vi "Lab Panel V4.90.vi"() -> ()   [LabVIEW 2013] (continued)
                    n1117 = Greater Or Equal?(x=w2162, y=w2155) -> (x >= y?=w2164:bool)
                    n1118 = case shown="True" w2164 {
                      tunnel: w2159 -> [w2174 _]
                      tunnel: w2158 -> [w2173 _]
                      tunnel: w2157 -> [w2172 _]
                      tunnel: w2156 -> [w2171 _]
                      frame True {
                        n1119 = stacked-sequence {
                          tunnel: w2174 -> [w2178 _]
                          tunnel: w2173 -> [w2176 w2182]
                          tunnel: w2172 -> [_ w2185]
                          tunnel: w2171 -> [w2175 _]
                          frame #0 {
                            n1120 = Build Array(w2176) -> (w2179:string[])
                            n1121 = Build Array(w2178) -> (w2177:dbl[])
                            n1122 = TDMS Write(0:w2175, 5:"TEST PASS", 7:w2179, 9:w2177) -> (15:w2181:errorcluster)  [unwired: 2 in, 3 out]
                            n1123 = local write "data file error"(w2181) -> ()
                          }
                          frame #1 {
                            n1124 = Bundle(cluster=w2185, "STATUS"=w2182) -> (w2183:T4)  [unwired: 2 in]
                            n1125 = local write "RESULT LAB02-1"(TRUE) -> ()
                            n1126 = local write "DISP LAB02-1"(w2183) -> ()
                          }
                        }
                      }
                      frame False {
                      }
                    }
                  }
                }
              }
              frame #3 {
                # "LAB02-2"
                n1127 = Less?(x=w2186, y=2) -> (x < y?=w2189:bool)
                n1128 = local read "DISP LAB02-2"() -> (w2191:T4)
                n1129 = Unbundle(w2191) -> ("STATUS"=w2192:string)  [unwired: 2 out]
                n1130 = Equal?(x=w2192, y="RUN") -> (x = y?=w2188:bool)
                n1131 = And(x=w2188, y=w2189) -> (x .and. y?=w2187:bool)
                n1132 = case shown="True" w2187 {
                  tunnel: w2191 -> [_ w2197]
                  tunnel: w2186 -> [_ w2201]
                  frame False {
                  }
                  frame True {
                    n1133 = local read "SET LAB02-2"() -> (w2203:T5)
                    n1134 = local read "TDMS LAB02-2"() -> (w2196:refnum<k34>)
                    n1135 = Unbundle(w2197) -> ("CYCLE"=w2202:dbl)  [unwired: 2 out]
                    n1136 = Unbundle(w2203) -> ("CYCLES"=w2194:dbl, "T-RISE mins"=w2200:dbl)  [unwired: 3 out]
                    n1137 = case shown="\"T-RISE TEST\"" w2201 {
                      tunnel: w2200 -> [_ _ w2210]
                      tunnel: [w2205 w2207 w2210] -> w2199
                      tunnel: w2194 -> [w2205 w2207 _]
                      tunnel: ["CHART PASS" "CYCLE PASS" "T-RISE PASS"] -> w2198
                      frame "CHART TEST", Default {
                      }
                      frame "CYCLE TEST" {
                      }
                      frame "T-RISE TEST" {
                      }
                    }
                    n1138 = Increment(x=w2194) -> (x+1=w2195:dbl)
                    n1139 = Greater Or Equal?(x=w2202, y=w2195) -> (x >= y?=w2204:bool)
                    n1140 = case shown="True" w2204 {
                      tunnel: w2199 -> [w2214 _]
                      tunnel: w2198 -> [w2213 _]
                      tunnel: w2197 -> [w2212 _]
                      tunnel: w2196 -> [w2211 _]
                      frame True {
                        n1141 = stacked-sequence {
                          tunnel: w2214 -> [w2218 _]
                          tunnel: w2213 -> [w2216 w2222]
                          tunnel: w2212 -> [_ w2225]
                          tunnel: w2211 -> [w2215 _]
                          frame #0 {
                            n1142 = Build Array(w2216) -> (w2219:string[])
                            n1143 = Build Array(w2218) -> (w2217:dbl[])
                            n1144 = TDMS Write(0:w2215, 5:"TEST PASS", 7:w2219, 9:w2217) -> (15:w2221:errorcluster)  [unwired: 2 in, 3 out]
                            n1145 = local write "data file error"(w2221) -> ()
                          }
                          frame #1 {
                            n1146 = Bundle(cluster=w2225, "STATUS"=w2222) -> (w2223:T4)  [unwired: 2 in]
                            n1147 = local write "RESULT LAB02-2"(TRUE) -> ()
                            n1148 = local write "DISP LAB02-2"(w2223) -> ()
                          }
                        }
                      }
                      frame False {
                      }
                    }
                  }
                }
              }
              frame #4 {
                # "LAB03-1"
                n1149 = Less?(x=w2226, y=2) -> (x < y?=w2229:bool)
                n1150 = local read "DISP LAB03-1"() -> (w2231:T4)
                n1151 = Unbundle(w2231) -> ("STATUS"=w2232:string)  [unwired: 2 out]
                n1152 = Equal?(x=w2232, y="RUN") -> (x = y?=w2228:bool)
                n1153 = And(x=w2228, y=w2229) -> (x .and. y?=w2227:bool)
                n1154 = case shown="True" w2227 {
                  tunnel: w2231 -> [_ w2237]
                  tunnel: w2226 -> [_ w2241]
                  frame False {
                  }
                  frame True {
                    n1155 = local read "SET LAB03-1"() -> (w2243:T5)
                    n1156 = local read "TDMS LAB03-1"() -> (w2236:refnum<k34>)
                    n1157 = Unbundle(w2237) -> ("CYCLE"=w2242:dbl)  [unwired: 2 out]
                    n1158 = Unbundle(w2243) -> ("CYCLES"=w2234:dbl, "T-RISE mins"=w2240:dbl)  [unwired: 3 out]
                    n1159 = case shown="\"T-RISE TEST\"" w2241 {
                      tunnel: w2240 -> [_ _ w2250]
                      tunnel: [w2245 w2247 w2250] -> w2239
                      tunnel: w2234 -> [w2245 w2247 _]
                      tunnel: ["CHART PASS" "CYCLE PASS" "T-RISE PASS"] -> w2238
                      frame "CHART TEST", Default {
                      }
                      frame "CYCLE TEST" {
                      }
                      frame "T-RISE TEST" {
                      }
                    }
                    n1160 = Increment(x=w2234) -> (x+1=w2235:dbl)
                    n1161 = Greater Or Equal?(x=w2242, y=w2235) -> (x >= y?=w2244:bool)
                    n1162 = case shown="True" w2244 {
                      tunnel: w2239 -> [w2254 _]
                      tunnel: w2238 -> [w2253 _]
                      tunnel: w2237 -> [w2252 _]
                      tunnel: w2236 -> [w2251 _]
                      frame True {
                        n1163 = stacked-sequence {
                          tunnel: w2254 -> [w2258 _]
                          tunnel: w2253 -> [w2256 w2262]
                          tunnel: w2252 -> [_ w2265]
                          tunnel: w2251 -> [w2255 _]
                          frame #0 {
                            n1164 = Build Array(w2256) -> (w2259:string[])
                            n1165 = Build Array(w2258) -> (w2257:dbl[])
                            n1166 = TDMS Write(0:w2255, 5:"TEST PASS", 7:w2259, 9:w2257) -> (15:w2261:errorcluster)  [unwired: 2 in, 3 out]
                            n1167 = local write "data file error"(w2261) -> ()
                          }
                          frame #1 {
                            n1168 = Bundle(cluster=w2265, "STATUS"=w2262) -> (w2263:T4)  [unwired: 2 in]
                            n1169 = local write "RESULT LAB03-1"(TRUE) -> ()
                            n1170 = local write "DISP LAB03-1"(w2263) -> ()
                          }
                        }
                      }
                      frame False {
                      }
                    }
                  }
                }
              }
              frame #5 {
                # "LAB03-2"
                n1171 = Less?(x=w2266, y=2) -> (x < y?=w2269:bool)
                n1172 = local read "DISP LAB03-2"() -> (w2271:T4)
                n1173 = Unbundle(w2271) -> ("STATUS"=w2272:string)  [unwired: 2 out]
                n1174 = Equal?(x=w2272, y="RUN") -> (x = y?=w2268:bool)
                n1175 = And(x=w2268, y=w2269) -> (x .and. y?=w2267:bool)
                n1176 = case shown="True" w2267 {
                  tunnel: w2271 -> [_ w2277]
                  tunnel: w2266 -> [_ w2281]
                  frame False {
                  }
                  frame True {
                    n1177 = local read "SET LAB03-2"() -> (w2283:T5)
                    n1178 = local read "TDMS LAB03-2"() -> (w2276:refnum<k34>)
                    n1179 = Unbundle(w2277) -> ("CYCLE"=w2282:dbl)  [unwired: 2 out]
                    n1180 = Unbundle(w2283) -> ("CYCLES"=w2274:dbl, "T-RISE mins"=w2280:dbl)  [unwired: 3 out]
                    n1181 = case shown="\"T-RISE TEST\"" w2281 {
                      tunnel: w2280 -> [_ _ w2290]
                      tunnel: [w2285 w2287 w2290] -> w2279
                      tunnel: w2274 -> [w2285 w2287 _]
                      tunnel: ["CHART PASS" "CYCLE PASS" "T-RISE PASS"] -> w2278
                      frame "CHART TEST", Default {
                      }
                      frame "CYCLE TEST" {
                      }
                      frame "T-RISE TEST" {
                      }
                    }
                    n1182 = Increment(x=w2274) -> (x+1=w2275:dbl)
                    n1183 = Greater Or Equal?(x=w2282, y=w2275) -> (x >= y?=w2284:bool)
                    n1184 = case shown="True" w2284 {
                      tunnel: w2279 -> [w2294 _]
                      tunnel: w2278 -> [w2293 _]
                      tunnel: w2277 -> [w2292 _]
                      tunnel: w2276 -> [w2291 _]
                      frame True {
                        n1185 = stacked-sequence {
                          tunnel: w2294 -> [w2298 _]
                          tunnel: w2293 -> [w2296 w2302]
                          tunnel: w2292 -> [_ w2305]
                          tunnel: w2291 -> [w2295 _]
                          frame #0 {
                            n1186 = Build Array(w2296) -> (w2299:string[])
                            n1187 = Build Array(w2298) -> (w2297:dbl[])
                            n1188 = TDMS Write(0:w2295, 5:"TEST PASS", 7:w2299, 9:w2297) -> (15:w2301:errorcluster)  [unwired: 2 in, 3 out]
                            n1189 = local write "data file error"(w2301) -> ()
                          }
                          frame #1 {
                            n1190 = Bundle(cluster=w2305, "STATUS"=w2302) -> (w2303:T4)  [unwired: 2 in]
                            n1191 = local write "RESULT LAB03-2"(TRUE) -> ()
                            n1192 = local write "DISP LAB03-2"(w2303) -> ()
                          }
                        }
                      }
                      frame False {
                      }
                    }
                  }
                }
              }
              frame #6 {
                # "LAB04-1"
                n1193 = Less?(x=w2306, y=2) -> (x < y?=w2309:bool)
                n1194 = local read "DISP LAB04-1"() -> (w2311:T4)
                n1195 = Unbundle(w2311) -> ("STATUS"=w2312:string)  [unwired: 2 out]
                n1196 = Equal?(x=w2312, y="RUN") -> (x = y?=w2308:bool)
                n1197 = And(x=w2308, y=w2309) -> (x .and. y?=w2307:bool)
                n1198 = case shown="True" w2307 {
                  tunnel: w2311 -> [_ w2317]
                  tunnel: w2306 -> [_ w2321]
                  frame False {
                  }
                  frame True {
                    n1199 = local read "SET LAB04-1"() -> (w2323:T5)
                    n1200 = local read "TDMS LAB04-1"() -> (w2316:refnum<k34>)
                    n1201 = Unbundle(w2317) -> ("CYCLE"=w2322:dbl)  [unwired: 2 out]
                    n1202 = Unbundle(w2323) -> ("CYCLES"=w2314:dbl, "T-RISE mins"=w2320:dbl)  [unwired: 3 out]
                    n1203 = case shown="\"T-RISE TEST\"" w2321 {
                      tunnel: w2320 -> [_ _ w2330]
                      tunnel: [w2325 w2327 w2330] -> w2319
                      tunnel: w2314 -> [w2325 w2327 _]
                      tunnel: ["CHART PASS" "CYCLE PASS" "T-RISE PASS"] -> w2318
                      frame "CHART TEST", Default {
                      }
                      frame "CYCLE TEST" {
                      }
                      frame "T-RISE TEST" {
                      }
                    }
                    n1204 = Increment(x=w2314) -> (x+1=w2315:dbl)
                    n1205 = Greater Or Equal?(x=w2322, y=w2315) -> (x >= y?=w2324:bool)
                    n1206 = case shown="True" w2324 {
                      tunnel: w2319 -> [w2334 _]
                      tunnel: w2318 -> [w2333 _]
                      tunnel: w2317 -> [w2332 _]
                      tunnel: w2316 -> [w2331 _]
                      frame True {
                        n1207 = stacked-sequence {
                          tunnel: w2334 -> [w2338 _]
                          tunnel: w2333 -> [w2336 w2342]
                          tunnel: w2332 -> [_ w2345]
                          tunnel: w2331 -> [w2335 _]
                          frame #0 {
                            n1208 = Build Array(w2336) -> (w2339:string[])
                            n1209 = Build Array(w2338) -> (w2337:dbl[])
                            n1210 = TDMS Write(0:w2335, 5:"TEST PASS", 7:w2339, 9:w2337) -> (15:w2341:errorcluster)  [unwired: 2 in, 3 out]
                            n1211 = local write "data file error"(w2341) -> ()
                          }
                          frame #1 {
                            n1212 = Bundle(cluster=w2345, "STATUS"=w2342) -> (w2343:T4)  [unwired: 2 in]
                            n1213 = local write "RESULT LAB04-1"(TRUE) -> ()
                            n1214 = local write "DISP LAB04-1"(w2343) -> ()
                          }
                        }
                      }
                      frame False {
                      }
                    }
                  }
                }
              }
              frame #7 {
                # "LAB04-2"
                n1215 = Less?(x=w2346, y=2) -> (x < y?=w2349:bool)
                n1216 = local read "DISP LAB04-2"() -> (w2351:T4)
                n1217 = Unbundle(w2351) -> ("STATUS"=w2352:string)  [unwired: 2 out]
                n1218 = Equal?(x=w2352, y="RUN") -> (x = y?=w2348:bool)
                n1219 = And(x=w2348, y=w2349) -> (x .and. y?=w2347:bool)
                n1220 = case shown="True" w2347 {
                  tunnel: w2351 -> [_ w2357]
                  tunnel: w2346 -> [_ w2361]
                  frame False {
                  }
                  frame True {
                    n1221 = local read "SET LAB04-2"() -> (w2363:T5)
                    n1222 = local read "TDMS LAB04-2"() -> (w2356:refnum<k34>)
                    n1223 = Unbundle(w2357) -> ("CYCLE"=w2362:dbl)  [unwired: 2 out]
                    n1224 = Unbundle(w2363) -> ("CYCLES"=w2354:dbl, "T-RISE mins"=w2360:dbl)  [unwired: 3 out]
                    n1225 = case shown="\"T-RISE TEST\"" w2361 {
                      tunnel: w2360 -> [_ _ w2370]
                      tunnel: [w2365 w2367 w2370] -> w2359
                      tunnel: w2354 -> [w2365 w2367 _]
                      tunnel: ["CHART PASS" "CYCLE PASS" "T-RISE PASS"] -> w2358
                      frame "CHART TEST", Default {
                      }
                      frame "CYCLE TEST" {
                      }
                      frame "T-RISE TEST" {
                      }
                    }
                    n1226 = Increment(x=w2354) -> (x+1=w2355:dbl)
                    n1227 = Greater Or Equal?(x=w2362, y=w2355) -> (x >= y?=w2364:bool)
                    n1228 = case shown="True" w2364 {
                      tunnel: w2359 -> [w2374 _]
                      tunnel: w2358 -> [w2373 _]
                      tunnel: w2357 -> [w2372 _]
                      tunnel: w2356 -> [w2371 _]
                      frame True {
                        n1229 = stacked-sequence {
                          tunnel: w2374 -> [w2378 _]
                          tunnel: w2373 -> [w2376 w2382]
                          tunnel: w2372 -> [_ w2385]
                          tunnel: w2371 -> [w2375 _]
                          frame #0 {
                            n1230 = Build Array(w2376) -> (w2379:string[])
                            n1231 = Build Array(w2378) -> (w2377:dbl[])
                            n1232 = TDMS Write(0:w2375, 5:"TEST PASS", 7:w2379, 9:w2377) -> (15:w2381:errorcluster)  [unwired: 2 in, 3 out]
                            n1233 = local write "data file error"(w2381) -> ()
                          }
                          frame #1 {
                            n1234 = Bundle(cluster=w2385, "STATUS"=w2382) -> (w2383:T4)  [unwired: 2 in]
                            n1235 = local write "RESULT LAB04-2"(TRUE) -> ()
                            n1236 = local write "DISP LAB04-2"(w2383) -> ()
                          }
                        }
                      }
                      frame False {
                      }
                    }
                  }
                }
              }
              frame #8 {
                # "LAB05-1"
                n1237 = Less?(x=w2386, y=2) -> (x < y?=w2389:bool)
                n1238 = local read "DISP LAB05-1"() -> (w2391:T4)
                n1239 = Unbundle(w2391) -> ("STATUS"=w2392:string)  [unwired: 2 out]
                n1240 = Equal?(x=w2392, y="RUN") -> (x = y?=w2388:bool)
                n1241 = And(x=w2388, y=w2389) -> (x .and. y?=w2387:bool)
                n1242 = case shown="True" w2387 {
                  tunnel: w2391 -> [_ w2397]
                  tunnel: w2386 -> [_ w2401]
                  frame False {
                  }
                  frame True {
                    n1243 = local read "SET LAB05-1"() -> (w2403:T5)
                    n1244 = local read "TDMS LAB05-1"() -> (w2396:refnum<k34>)
                    n1245 = Unbundle(w2397) -> ("CYCLE"=w2402:dbl)  [unwired: 2 out]
                    n1246 = Unbundle(w2403) -> ("CYCLES"=w2394:dbl, "T-RISE mins"=w2400:dbl)  [unwired: 3 out]
                    n1247 = case shown="\"T-RISE TEST\"" w2401 {
                      tunnel: w2400 -> [_ _ w2410]
                      tunnel: [w2405 w2407 w2410] -> w2399
                      tunnel: w2394 -> [w2405 w2407 _]
                      tunnel: ["CHART PASS" "CYCLE PASS" "T-RISE PASS"] -> w2398
                      frame "CHART TEST", Default {
                      }
                      frame "CYCLE TEST" {
                      }
                      frame "T-RISE TEST" {
                      }
                    }
                    n1248 = Increment(x=w2394) -> (x+1=w2395:dbl)
                    n1249 = Greater Or Equal?(x=w2402, y=w2395) -> (x >= y?=w2404:bool)
                    n1250 = case shown="True" w2404 {
                      tunnel: w2399 -> [w2414 _]
                      tunnel: w2398 -> [w2413 _]
                      tunnel: w2397 -> [w2412 _]
                      tunnel: w2396 -> [w2411 _]
                      frame True {
                        n1251 = stacked-sequence {
                          tunnel: w2414 -> [w2418 _]
                          tunnel: w2413 -> [w2416 w2422]
                          tunnel: w2412 -> [_ w2425]
                          tunnel: w2411 -> [w2415 _]
                          frame #0 {
                            n1252 = Build Array(w2416) -> (w2419:string[])
                            n1253 = Build Array(w2418) -> (w2417:dbl[])
                            n1254 = TDMS Write(0:w2415, 5:"TEST PASS", 7:w2419, 9:w2417) -> (15:w2421:errorcluster)  [unwired: 2 in, 3 out]
                            n1255 = local write "data file error"(w2421) -> ()
                          }
                          frame #1 {
                            n1256 = Bundle(cluster=w2425, "STATUS"=w2422) -> (w2423:T4)  [unwired: 2 in]
                            n1257 = local write "RESULT LAB05-1"(TRUE) -> ()
                            n1258 = local write "DISP LAB05-1"(w2423) -> ()
                          }
                        }
                      }
                      frame False {
                      }
                    }
                  }
                }
              }
              frame #9 {
                # "LAB05-2"
                n1259 = Less?(x=w2426, y=2) -> (x < y?=w2429:bool)
                n1260 = local read "DISP LAB05-2"() -> (w2431:T4)
                n1261 = Unbundle(w2431) -> ("STATUS"=w2432:string)  [unwired: 2 out]
                n1262 = Equal?(x=w2432, y="RUN") -> (x = y?=w2428:bool)
                n1263 = And(x=w2428, y=w2429) -> (x .and. y?=w2427:bool)
                n1264 = case shown="True" w2427 {
                  tunnel: w2431 -> [_ w2437]
                  tunnel: w2426 -> [_ w2441]
                  frame False {
                  }
                  frame True {
                    n1265 = local read "SET LAB05-2"() -> (w2443:T5)
                    n1266 = local read "TDMS LAB05-2"() -> (w2436:refnum<k34>)
                    n1267 = Unbundle(w2437) -> ("CYCLE"=w2442:dbl)  [unwired: 2 out]
                    n1268 = Unbundle(w2443) -> ("CYCLES"=w2434:dbl, "T-RISE mins"=w2440:dbl)  [unwired: 3 out]
                    n1269 = case shown="\"T-RISE TEST\"" w2441 {
                      tunnel: w2440 -> [_ _ w2450]
                      tunnel: [w2445 w2447 w2450] -> w2439
                      tunnel: w2434 -> [w2445 w2447 _]
                      tunnel: ["CHART PASS" "CYCLE PASS" "T-RISE PASS"] -> w2438
                      frame "CHART TEST", Default {
                      }
                      frame "CYCLE TEST" {
                      }
                      frame "T-RISE TEST" {
                      }
                    }
                    n1270 = Increment(x=w2434) -> (x+1=w2435:dbl)
                    n1271 = Greater Or Equal?(x=w2442, y=w2435) -> (x >= y?=w2444:bool)
                    n1272 = case shown="True" w2444 {
                      tunnel: w2439 -> [w2454 _]
                      tunnel: w2438 -> [w2453 _]
                      tunnel: w2437 -> [w2452 _]
                      tunnel: w2436 -> [w2451 _]
                      frame True {
                        n1273 = stacked-sequence {
                          tunnel: w2454 -> [w2458 _]
                          tunnel: w2453 -> [w2456 w2462]
                          tunnel: w2452 -> [_ w2465]
                          tunnel: w2451 -> [w2455 _]
                          frame #0 {
                            n1274 = Build Array(w2456) -> (w2459:string[])
                            n1275 = Build Array(w2458) -> (w2457:dbl[])
                            n1276 = TDMS Write(0:w2455, 5:"TEST PASS", 7:w2459, 9:w2457) -> (15:w2461:errorcluster)  [unwired: 2 in, 3 out]
                            n1277 = local write "data file error"(w2461) -> ()
                          }
                          frame #1 {
                            n1278 = Bundle(cluster=w2465, "STATUS"=w2462) -> (w2463:T4)  [unwired: 2 in]
                            n1279 = local write "RESULT LAB05-2"(TRUE) -> ()
                            n1280 = local write "DISP LAB05-2"(w2463) -> ()
                          }
                        }
                      }
                      frame False {
                      }
                    }
                  }
                }
              }
            }
          }
          frame #5 {
            # "check if test cycles reached for temperature rise test"
            n1281 = stacked-sequence {
              tunnel: w2495 -> [_ _ _ _ _ _ _ _ _ _]
              tunnel: w2494 -> [_ _ _ _ _ _ _ _ _ _]
              tunnel: w2493 -> [_ _ _ _ _ _ _ _ _ _]
              tunnel: w2492 -> [_ _ _ _ _ _ _ _ _ _]
              tunnel: w2491 -> [_ _ _ _ _ _ _ _ _ _]
              tunnel: w2490 -> [_ _ _ _ _ _ _ _ _ _]
              tunnel: w2489 -> [_ _ _ _ _ _ _ _ _ _]
              tunnel: w2488 -> [_ _ _ _ _ _ _ _ _ _]
              tunnel: w2487 -> [_ _ _ _ _ _ _ _ _ _]
              tunnel: w2486 -> [_ _ _ _ _ _ _ _ _ _]
              tunnel: w2485 -> [w2501 _ _ _ _ _ _ _ _ _]
              tunnel: w2475 -> [w2496 _ _ _ _ _ _ _ _ _]
              tunnel: w2484 -> [_ w2527 _ _ _ _ _ _ _ _]
              tunnel: w2483 -> [_ _ w2557 _ _ _ _ _ _ _]
              tunnel: w2482 -> [_ _ _ w2587 _ _ _ _ _ _]
              tunnel: w2481 -> [_ _ _ _ w2617 _ _ _ _ _]
              tunnel: w2480 -> [_ _ _ _ _ w2647 _ _ _ _]
              tunnel: w2479 -> [_ _ _ _ _ _ w2677 _ _ _]
              tunnel: w2478 -> [_ _ _ _ _ _ _ w2707 _ _]
              tunnel: w2477 -> [_ _ _ _ _ _ _ _ w2737 _]
              tunnel: w2476 -> [_ _ _ _ _ _ _ _ _ w2767]
              tunnel: w2474 -> [_ w2526 _ _ _ _ _ _ _ _]
              tunnel: w2473 -> [_ _ w2556 _ _ _ _ _ _ _]
              tunnel: w2472 -> [_ _ _ w2586 _ _ _ _ _ _]
              tunnel: w2471 -> [_ _ _ _ w2616 _ _ _ _ _]
              tunnel: w2470 -> [_ _ _ _ _ w2646 _ _ _ _]
              tunnel: w2469 -> [_ _ _ _ _ _ w2676 _ _ _]
              tunnel: w2468 -> [_ _ _ _ _ _ _ w2706 _ _]
              tunnel: w2467 -> [_ _ _ _ _ _ _ _ w2736 _]
              tunnel: w2466 -> [_ _ _ _ _ _ _ _ _ w2766]
              frame #0 {
                # "LAB01-1"
                n1282 = Equal?(x=w2501, y=2) -> (x = y?=w2499:bool)
                n1283 = local read "DISP LAB01-1"() -> (w2502:T4)
                n1284 = Unbundle(w2502) -> ("STATUS"=w2503:string)  [unwired: 2 out]
                n1285 = Equal?(x=w2503, y="RUN") -> (x = y?=w2498:bool)
                n1286 = And(x=w2498, y=w2499) -> (x .and. y?=w2497:bool)
                n1287 = case shown="True" w2497 {
                  tunnel: w2502 -> [_ w2506]
                  tunnel: w2496 -> [_ w2509]
                  frame False {
                  }
                  frame True {
                    n1288 = local read "SET LAB01-1"() -> (w2508:T5)
                    n1289 = local read "TDMS LAB01-1"() -> (w2505:refnum<k34>)
                    n1290 = Unbundle(w2506) -> ("CYCLE"=w2510:dbl)  [unwired: 2 out]
                    n1291 = Unbundle(w2508) -> ("T-RISE mins"=w2507:dbl)  [unwired: 4 out]
                    n1292 = Greater Or Equal?(x=w2510, y=w2509) -> (x >= y?=w2511:bool)
                    n1293 = case shown="True" w2511 {
                      tunnel: w2507 -> [w2514 _]
                      tunnel: w2506 -> [w2513 _]
                      tunnel: w2505 -> [w2512 _]
                      frame True {
                        n1294 = stacked-sequence {
                          tunnel: w2514 -> [w2517 _]
                          tunnel: w2513 -> [_ w2522]
                          tunnel: w2512 -> [w2515 _]
                          frame #0 {
                            n1295 = Build Array("T-RISE") -> (w2519:string[])
                            n1296 = Build Array(w2517) -> (w2518:dbl[])
                            n1297 = TDMS Write(0:w2515, 5:"TEST PASS", 7:w2519, 9:w2518) -> (15:w2521:errorcluster)  [unwired: 2 in, 3 out]
                            n1298 = local write "data file error"(w2521) -> ()
                          }
                          frame #1 {
                            n1299 = Bundle(cluster=w2522, "STATUS"="T-RISE PASS") -> (w2524:T4)  [unwired: 2 in]
                            n1300 = local write "RESULT LAB01-1"(TRUE) -> ()
                            n1301 = local write "DISP LAB01-1"(w2524) -> ()
                          }
                        }
                      }
                      frame False {
                      }
                    }
                  }
                }
              }
              frame #1 {
                # "LAB01-2"
                n1302 = Equal?(x=w2527, y=2) -> (x = y?=w2530:bool)
                n1303 = local read "DISP LAB01-2"() -> (w2532:T4)
                n1304 = Unbundle(w2532) -> ("STATUS"=w2533:string)  [unwired: 2 out]
                n1305 = Equal?(x=w2533, y="RUN") -> (x = y?=w2529:bool)
                n1306 = And(x=w2529, y=w2530) -> (x .and. y?=w2528:bool)
                n1307 = case shown="True" w2528 {
                  tunnel: w2532 -> [_ w2536]
                  tunnel: w2526 -> [_ w2539]
                  frame False {
                  }
                  frame True {
                    n1308 = local read "SET LAB01-2"() -> (w2538:T5)
                    n1309 = local read "TDMS LAB01-2"() -> (w2535:refnum<k34>)
                    n1310 = Unbundle(w2536) -> ("CYCLE"=w2540:dbl)  [unwired: 2 out]
                    n1311 = Unbundle(w2538) -> ("T-RISE mins"=w2537:dbl)  [unwired: 4 out]
                    n1312 = Greater Or Equal?(x=w2540, y=w2539) -> (x >= y?=w2541:bool)
                    n1313 = case shown="True" w2541 {
                      tunnel: w2537 -> [w2544 _]
                      tunnel: w2536 -> [w2543 _]
                      tunnel: w2535 -> [w2542 _]
                      frame True {
                        n1314 = stacked-sequence {
                          tunnel: w2544 -> [w2547 _]
                          tunnel: w2543 -> [_ w2552]
                          tunnel: w2542 -> [w2545 _]
                          frame #0 {
                            n1315 = Build Array("T-RISE") -> (w2549:string[])
                            n1316 = Build Array(w2547) -> (w2548:dbl[])
                            n1317 = TDMS Write(0:w2545, 5:"TEST PASS", 7:w2549, 9:w2548) -> (15:w2551:errorcluster)  [unwired: 2 in, 3 out]
                            n1318 = local write "data file error"(w2551) -> ()
                          }
                          frame #1 {
                            n1319 = Bundle(cluster=w2552, "STATUS"="T-RISE PASS") -> (w2554:T4)  [unwired: 2 in]
                            n1320 = local write "RESULT LAB01-2"(TRUE) -> ()
                            n1321 = local write "DISP LAB01-2"(w2554) -> ()
                          }
                        }
                      }
                      frame False {
                      }
                    }
                  }
                }
              }
              frame #2 {
                # "LAB02-1"
                n1322 = Equal?(x=w2557, y=2) -> (x = y?=w2560:bool)
                n1323 = local read "DISP LAB02-1"() -> (w2562:T4)
                n1324 = Unbundle(w2562) -> ("STATUS"=w2563:string)  [unwired: 2 out]
                n1325 = Equal?(x=w2563, y="RUN") -> (x = y?=w2559:bool)
                n1326 = And(x=w2559, y=w2560) -> (x .and. y?=w2558:bool)
                n1327 = case shown="True" w2558 {
                  tunnel: w2562 -> [_ w2566]
                  tunnel: w2556 -> [_ w2569]
                  frame False {
                  }
                  frame True {
                    n1328 = local read "SET LAB02-1"() -> (w2568:T5)
                    n1329 = local read "TDMS LAB02-1"() -> (w2565:refnum<k34>)
                    n1330 = Unbundle(w2566) -> ("CYCLE"=w2570:dbl)  [unwired: 2 out]
                    n1331 = Unbundle(w2568) -> ("T-RISE mins"=w2567:dbl)  [unwired: 4 out]
                    n1332 = Greater Or Equal?(x=w2570, y=w2569) -> (x >= y?=w2571:bool)
                    n1333 = case shown="True" w2571 {
                      tunnel: w2567 -> [w2574 _]
                      tunnel: w2566 -> [w2573 _]
                      tunnel: w2565 -> [w2572 _]
                      frame True {
                        n1334 = stacked-sequence {
                          tunnel: w2574 -> [w2577 _]
                          tunnel: w2573 -> [_ w2582]
                          tunnel: w2572 -> [w2575 _]
                          frame #0 {
                            n1335 = Build Array("T-RISE") -> (w2579:string[])
                            n1336 = Build Array(w2577) -> (w2578:dbl[])
                            n1337 = TDMS Write(0:w2575, 5:"TEST PASS", 7:w2579, 9:w2578) -> (15:w2581:errorcluster)  [unwired: 2 in, 3 out]
                            n1338 = local write "data file error"(w2581) -> ()
                          }
                          frame #1 {
                            n1339 = Bundle(cluster=w2582, "STATUS"="T-RISE PASS") -> (w2584:T4)  [unwired: 2 in]
                            n1340 = local write "RESULT LAB02-1"(TRUE) -> ()
                            n1341 = local write "DISP LAB02-1"(w2584) -> ()
                          }
                        }
                      }
                      frame False {
                      }
                    }
                  }
                }
              }
              frame #3 {
                # "LAB02-2"
                n1342 = Equal?(x=w2587, y=2) -> (x = y?=w2590:bool)
                n1343 = local read "DISP LAB02-2"() -> (w2592:T4)
                n1344 = Unbundle(w2592) -> ("STATUS"=w2593:string)  [unwired: 2 out]
                n1345 = Equal?(x=w2593, y="RUN") -> (x = y?=w2589:bool)
                n1346 = And(x=w2589, y=w2590) -> (x .and. y?=w2588:bool)
                n1347 = case shown="True" w2588 {
                  tunnel: w2592 -> [_ w2596]
                  tunnel: w2586 -> [_ w2599]
                  frame False {
                  }
                  frame True {
                    n1348 = local read "SET LAB02-2"() -> (w2598:T5)
                    n1349 = local read "TDMS LAB02-2"() -> (w2595:refnum<k34>)
                    n1350 = Unbundle(w2596) -> ("CYCLE"=w2600:dbl)  [unwired: 2 out]
                    n1351 = Unbundle(w2598) -> ("T-RISE mins"=w2597:dbl)  [unwired: 4 out]
                    n1352 = Greater Or Equal?(x=w2600, y=w2599) -> (x >= y?=w2601:bool)
                    n1353 = case shown="True" w2601 {
                      tunnel: w2597 -> [w2604 _]
                      tunnel: w2596 -> [w2603 _]
                      tunnel: w2595 -> [w2602 _]
                      frame True {
                        n1354 = stacked-sequence {
                          tunnel: w2604 -> [w2607 _]
                          tunnel: w2603 -> [_ w2612]
                          tunnel: w2602 -> [w2605 _]
                          frame #0 {
                            n1355 = Build Array("T-RISE") -> (w2609:string[])
                            n1356 = Build Array(w2607) -> (w2608:dbl[])
                            n1357 = TDMS Write(0:w2605, 5:"TEST PASS", 7:w2609, 9:w2608) -> (15:w2611:errorcluster)  [unwired: 2 in, 3 out]
                            n1358 = local write "data file error"(w2611) -> ()
                          }
                          frame #1 {
                            n1359 = Bundle(cluster=w2612, "STATUS"="T-RISE PASS") -> (w2614:T4)  [unwired: 2 in]
                            n1360 = local write "RESULT LAB02-2"(TRUE) -> ()
                            n1361 = local write "DISP LAB02-2"(w2614) -> ()
                          }
                        }
                      }
                      frame False {
                      }
                    }
                  }
                }
              }
              frame #4 {
                # "LAB03-1"
                n1362 = Equal?(x=w2617, y=2) -> (x = y?=w2620:bool)
                n1363 = local read "DISP LAB03-1"() -> (w2622:T4)
                n1364 = Unbundle(w2622) -> ("STATUS"=w2623:string)  [unwired: 2 out]
                n1365 = Equal?(x=w2623, y="RUN") -> (x = y?=w2619:bool)
                n1366 = And(x=w2619, y=w2620) -> (x .and. y?=w2618:bool)
                n1367 = case shown="True" w2618 {
                  tunnel: w2622 -> [_ w2626]
                  tunnel: w2616 -> [_ w2629]
                  frame False {
                  }
                  frame True {
                    n1368 = local read "SET LAB03-1"() -> (w2628:T5)
                    n1369 = local read "TDMS LAB03-1"() -> (w2625:refnum<k34>)
                    n1370 = Unbundle(w2626) -> ("CYCLE"=w2630:dbl)  [unwired: 2 out]
                    n1371 = Unbundle(w2628) -> ("T-RISE mins"=w2627:dbl)  [unwired: 4 out]
                    n1372 = Greater Or Equal?(x=w2630, y=w2629) -> (x >= y?=w2631:bool)
                    n1373 = case shown="True" w2631 {
                      tunnel: w2627 -> [w2634 _]
                      tunnel: w2626 -> [w2633 _]
                      tunnel: w2625 -> [w2632 _]
                      frame True {
                        n1374 = stacked-sequence {
                          tunnel: w2634 -> [w2637 _]
                          tunnel: w2633 -> [_ w2642]
                          tunnel: w2632 -> [w2635 _]
                          frame #0 {
                            n1375 = Build Array("T-RISE") -> (w2639:string[])
                            n1376 = Build Array(w2637) -> (w2638:dbl[])
                            n1377 = TDMS Write(0:w2635, 5:"TEST PASS", 7:w2639, 9:w2638) -> (15:w2641:errorcluster)  [unwired: 2 in, 3 out]
                            n1378 = local write "data file error"(w2641) -> ()
                          }
                          frame #1 {
                            n1379 = Bundle(cluster=w2642, "STATUS"="T-RISE PASS") -> (w2644:T4)  [unwired: 2 in]
                            n1380 = local write "RESULT LAB03-1"(TRUE) -> ()
                            n1381 = local write "DISP LAB03-1"(w2644) -> ()
                          }
                        }
                      }
                      frame False {
                      }
                    }
                  }
                }
              }
              frame #5 {
                # "LAB03-2"
                n1382 = Equal?(x=w2647, y=2) -> (x = y?=w2650:bool)
                n1383 = local read "DISP LAB03-2"() -> (w2652:T4)
                n1384 = Unbundle(w2652) -> ("STATUS"=w2653:string)  [unwired: 2 out]
                n1385 = Equal?(x=w2653, y="RUN") -> (x = y?=w2649:bool)
                n1386 = And(x=w2649, y=w2650) -> (x .and. y?=w2648:bool)
                n1387 = case shown="True" w2648 {
                  tunnel: w2652 -> [_ w2656]
                  tunnel: w2646 -> [_ w2659]
                  frame False {
                  }
                  frame True {
                    n1388 = local read "SET LAB03-2"() -> (w2658:T5)
                    n1389 = local read "TDMS LAB03-2"() -> (w2655:refnum<k34>)
                    n1390 = Unbundle(w2656) -> ("CYCLE"=w2660:dbl)  [unwired: 2 out]
                    n1391 = Unbundle(w2658) -> ("T-RISE mins"=w2657:dbl)  [unwired: 4 out]
                    n1392 = Greater Or Equal?(x=w2660, y=w2659) -> (x >= y?=w2661:bool)
                    n1393 = case shown="True" w2661 {
                      tunnel: w2657 -> [w2664 _]
                      tunnel: w2656 -> [w2663 _]
                      tunnel: w2655 -> [w2662 _]
                      frame True {
                        n1394 = stacked-sequence {
                          tunnel: w2664 -> [w2667 _]
                          tunnel: w2663 -> [_ w2672]
                          tunnel: w2662 -> [w2665 _]
                          frame #0 {
                            n1395 = Build Array("T-RISE") -> (w2669:string[])
                            n1396 = Build Array(w2667) -> (w2668:dbl[])
                            n1397 = TDMS Write(0:w2665, 5:"TEST PASS", 7:w2669, 9:w2668) -> (15:w2671:errorcluster)  [unwired: 2 in, 3 out]
                            n1398 = local write "data file error"(w2671) -> ()
                          }
                          frame #1 {
                            n1399 = Bundle(cluster=w2672, "STATUS"="T-RISE PASS") -> (w2674:T4)  [unwired: 2 in]
                            n1400 = local write "RESULT LAB03-2"(TRUE) -> ()
                            n1401 = local write "DISP LAB03-2"(w2674) -> ()
                          }
                        }
                      }
                      frame False {
                      }
                    }
                  }
                }
              }
              frame #6 {
                # "LAB04-1"
                n1402 = Equal?(x=w2677, y=2) -> (x = y?=w2680:bool)
                n1403 = local read "DISP LAB04-1"() -> (w2682:T4)
                n1404 = Unbundle(w2682) -> ("STATUS"=w2683:string)  [unwired: 2 out]
                n1405 = Equal?(x=w2683, y="RUN") -> (x = y?=w2679:bool)
                n1406 = And(x=w2679, y=w2680) -> (x .and. y?=w2678:bool)
                n1407 = case shown="True" w2678 {
                  tunnel: w2682 -> [_ w2686]
                  tunnel: w2676 -> [_ w2689]
                  frame False {
                  }
                  frame True {
                    n1408 = local read "SET LAB04-1"() -> (w2688:T5)
                    n1409 = local read "TDMS LAB04-1"() -> (w2685:refnum<k34>)
                    n1410 = Unbundle(w2686) -> ("CYCLE"=w2690:dbl)  [unwired: 2 out]
                    n1411 = Unbundle(w2688) -> ("T-RISE mins"=w2687:dbl)  [unwired: 4 out]
                    n1412 = Greater Or Equal?(x=w2690, y=w2689) -> (x >= y?=w2691:bool)
                    n1413 = case shown="True" w2691 {
                      tunnel: w2687 -> [w2694 _]
                      tunnel: w2686 -> [w2693 _]
                      tunnel: w2685 -> [w2692 _]
                      frame True {
                        n1414 = stacked-sequence {
                          tunnel: w2694 -> [w2697 _]
                          tunnel: w2693 -> [_ w2702]
                          tunnel: w2692 -> [w2695 _]
                          frame #0 {
                            n1415 = Build Array("T-RISE") -> (w2699:string[])
                            n1416 = Build Array(w2697) -> (w2698:dbl[])
                            n1417 = TDMS Write(0:w2695, 5:"TEST PASS", 7:w2699, 9:w2698) -> (15:w2701:errorcluster)  [unwired: 2 in, 3 out]
                            n1418 = local write "data file error"(w2701) -> ()
                          }
                          frame #1 {
                            n1419 = Bundle(cluster=w2702, "STATUS"="T-RISE PASS") -> (w2704:T4)  [unwired: 2 in]
                            n1420 = local write "RESULT LAB04-1"(TRUE) -> ()
                            n1421 = local write "DISP LAB04-1"(w2704) -> ()
                          }
                        }
                      }
                      frame False {
                      }
                    }
                  }
                }
              }
              frame #7 {
                # "LAB04-2"
                n1422 = Equal?(x=w2707, y=2) -> (x = y?=w2710:bool)
                n1423 = local read "DISP LAB04-2"() -> (w2712:T4)
                n1424 = Unbundle(w2712) -> ("STATUS"=w2713:string)  [unwired: 2 out]
                n1425 = Equal?(x=w2713, y="RUN") -> (x = y?=w2709:bool)
                n1426 = And(x=w2709, y=w2710) -> (x .and. y?=w2708:bool)
                n1427 = case shown="True" w2708 {
                  tunnel: w2712 -> [_ w2716]
                  tunnel: w2706 -> [_ w2719]
                  frame False {
                  }
                  frame True {
                    n1428 = local read "SET LAB04-2"() -> (w2718:T5)
                    n1429 = local read "TDMS LAB04-2"() -> (w2715:refnum<k34>)
                    n1430 = Unbundle(w2716) -> ("CYCLE"=w2720:dbl)  [unwired: 2 out]
                    n1431 = Unbundle(w2718) -> ("T-RISE mins"=w2717:dbl)  [unwired: 4 out]
                    n1432 = Greater Or Equal?(x=w2720, y=w2719) -> (x >= y?=w2721:bool)
                    n1433 = case shown="True" w2721 {
                      tunnel: w2717 -> [w2724 _]
                      tunnel: w2716 -> [w2723 _]
                      tunnel: w2715 -> [w2722 _]
                      frame True {
                        n1434 = stacked-sequence {
                          tunnel: w2724 -> [w2727 _]
                          tunnel: w2723 -> [_ w2732]
                          tunnel: w2722 -> [w2725 _]
                          frame #0 {
                            n1435 = Build Array("T-RISE") -> (w2729:string[])
                            n1436 = Build Array(w2727) -> (w2728:dbl[])
                            n1437 = TDMS Write(0:w2725, 5:"TEST PASS", 7:w2729, 9:w2728) -> (15:w2731:errorcluster)  [unwired: 2 in, 3 out]
                            n1438 = local write "data file error"(w2731) -> ()
                          }
                          frame #1 {
                            n1439 = Bundle(cluster=w2732, "STATUS"="T-RISE PASS") -> (w2734:T4)  [unwired: 2 in]
                            n1440 = local write "RESULT LAB04-2"(TRUE) -> ()
                            n1441 = local write "DISP LAB04-2"(w2734) -> ()
                          }
                        }
                      }
                      frame False {
                      }
                    }
                  }
                }
              }
              frame #8 {
                # "LAB05-1"
                n1442 = Equal?(x=w2737, y=2) -> (x = y?=w2740:bool)
                n1443 = local read "DISP LAB05-1"() -> (w2742:T4)
                n1444 = Unbundle(w2742) -> ("STATUS"=w2743:string)  [unwired: 2 out]
                n1445 = Equal?(x=w2743, y="RUN") -> (x = y?=w2739:bool)
                n1446 = And(x=w2739, y=w2740) -> (x .and. y?=w2738:bool)
                n1447 = case shown="True" w2738 {
                  tunnel: w2742 -> [_ w2746]
                  tunnel: w2736 -> [_ w2749]
                  frame False {
                  }
                  frame True {
                    n1448 = local read "SET LAB05-1"() -> (w2748:T5)
                    n1449 = local read "TDMS LAB05-1"() -> (w2745:refnum<k34>)
                    n1450 = Unbundle(w2746) -> ("CYCLE"=w2750:dbl)  [unwired: 2 out]
                    n1451 = Unbundle(w2748) -> ("T-RISE mins"=w2747:dbl)  [unwired: 4 out]
                    n1452 = Greater Or Equal?(x=w2750, y=w2749) -> (x >= y?=w2751:bool)
                    n1453 = case shown="True" w2751 {
                      tunnel: w2747 -> [w2754 _]
                      tunnel: w2746 -> [w2753 _]
                      tunnel: w2745 -> [w2752 _]
                      frame True {
                        n1454 = stacked-sequence {
                          tunnel: w2754 -> [w2757 _]
                          tunnel: w2753 -> [_ w2762]
                          tunnel: w2752 -> [w2755 _]
                          frame #0 {
                            n1455 = Build Array("T-RISE") -> (w2759:string[])
                            n1456 = Build Array(w2757) -> (w2758:dbl[])
                            n1457 = TDMS Write(0:w2755, 5:"TEST PASS", 7:w2759, 9:w2758) -> (15:w2761:errorcluster)  [unwired: 2 in, 3 out]
                            n1458 = local write "data file error"(w2761) -> ()
                          }
                          frame #1 {
                            n1459 = Bundle(cluster=w2762, "STATUS"="T-RISE PASS") -> (w2764:T4)  [unwired: 2 in]
                            n1460 = local write "RESULT LAB05-1"(TRUE) -> ()
                            n1461 = local write "DISP LAB05-1"(w2764) -> ()
                          }
                        }
                      }
                      frame False {
                      }
                    }
                  }
                }
              }
              frame #9 {
                # "LAB05-2"
                n1462 = Equal?(x=w2767, y=2) -> (x = y?=w2770:bool)
                n1463 = local read "DISP LAB05-2"() -> (w2772:T4)
                n1464 = Unbundle(w2772) -> ("STATUS"=w2773:string)  [unwired: 2 out]
                n1465 = Equal?(x=w2773, y="RUN") -> (x = y?=w2769:bool)
                n1466 = And(x=w2769, y=w2770) -> (x .and. y?=w2768:bool)
                n1467 = case shown="True" w2768 {
                  tunnel: w2772 -> [_ w2776]
                  tunnel: w2766 -> [_ w2779]
                  frame False {
                  }
                  frame True {
                    n1468 = local read "SET LAB05-2"() -> (w2778:T5)
                    n1469 = local read "TDMS LAB05-2"() -> (w2775:refnum<k34>)
                    n1470 = Unbundle(w2776) -> ("CYCLE"=w2780:dbl)  [unwired: 2 out]
                    n1471 = Unbundle(w2778) -> ("T-RISE mins"=w2777:dbl)  [unwired: 4 out]
                    n1472 = Greater Or Equal?(x=w2780, y=w2779) -> (x >= y?=w2781:bool)
                    n1473 = case shown="True" w2781 {
                      tunnel: w2777 -> [w2784 _]
                      tunnel: w2776 -> [w2783 _]
                      tunnel: w2775 -> [w2782 _]
                      frame True {
                        n1474 = stacked-sequence {
                          tunnel: w2784 -> [w2787 _]
                          tunnel: w2783 -> [_ w2792]
                          tunnel: w2782 -> [w2785 _]
                          frame #0 {
                            n1475 = Build Array("T-RISE") -> (w2789:string[])
                            n1476 = Build Array(w2787) -> (w2788:dbl[])
                            n1477 = TDMS Write(0:w2785, 5:"TEST PASS", 7:w2789, 9:w2788) -> (15:w2791:errorcluster)  [unwired: 2 in, 3 out]
                            n1478 = local write "data file error"(w2791) -> ()
                          }
                          frame #1 {
                            n1479 = Bundle(cluster=w2792, "STATUS"="T-RISE PASS") -> (w2794:T4)  [unwired: 2 in]
